vi "HXG2_Fluid-Averages.vi"(8 "error in (no error)":errorcluster, 9 "Analog DATA In":T3, 10 "BoolSelection In":T2, 11 "CalcValues":T1) -> (0 "error out":errorcluster, 3 "Calculated Values":T1)   [LabVIEW 2012]
doc: "This VI will average all air side and glycol side input temperatures based on boolean selections of what sensors to use."
uses:
  Controls/HXG2_Calculated.ctl
  Controls/HXG2_AnalogIn.ctl
  Controls/HXG2_BooleanSelections.ctl
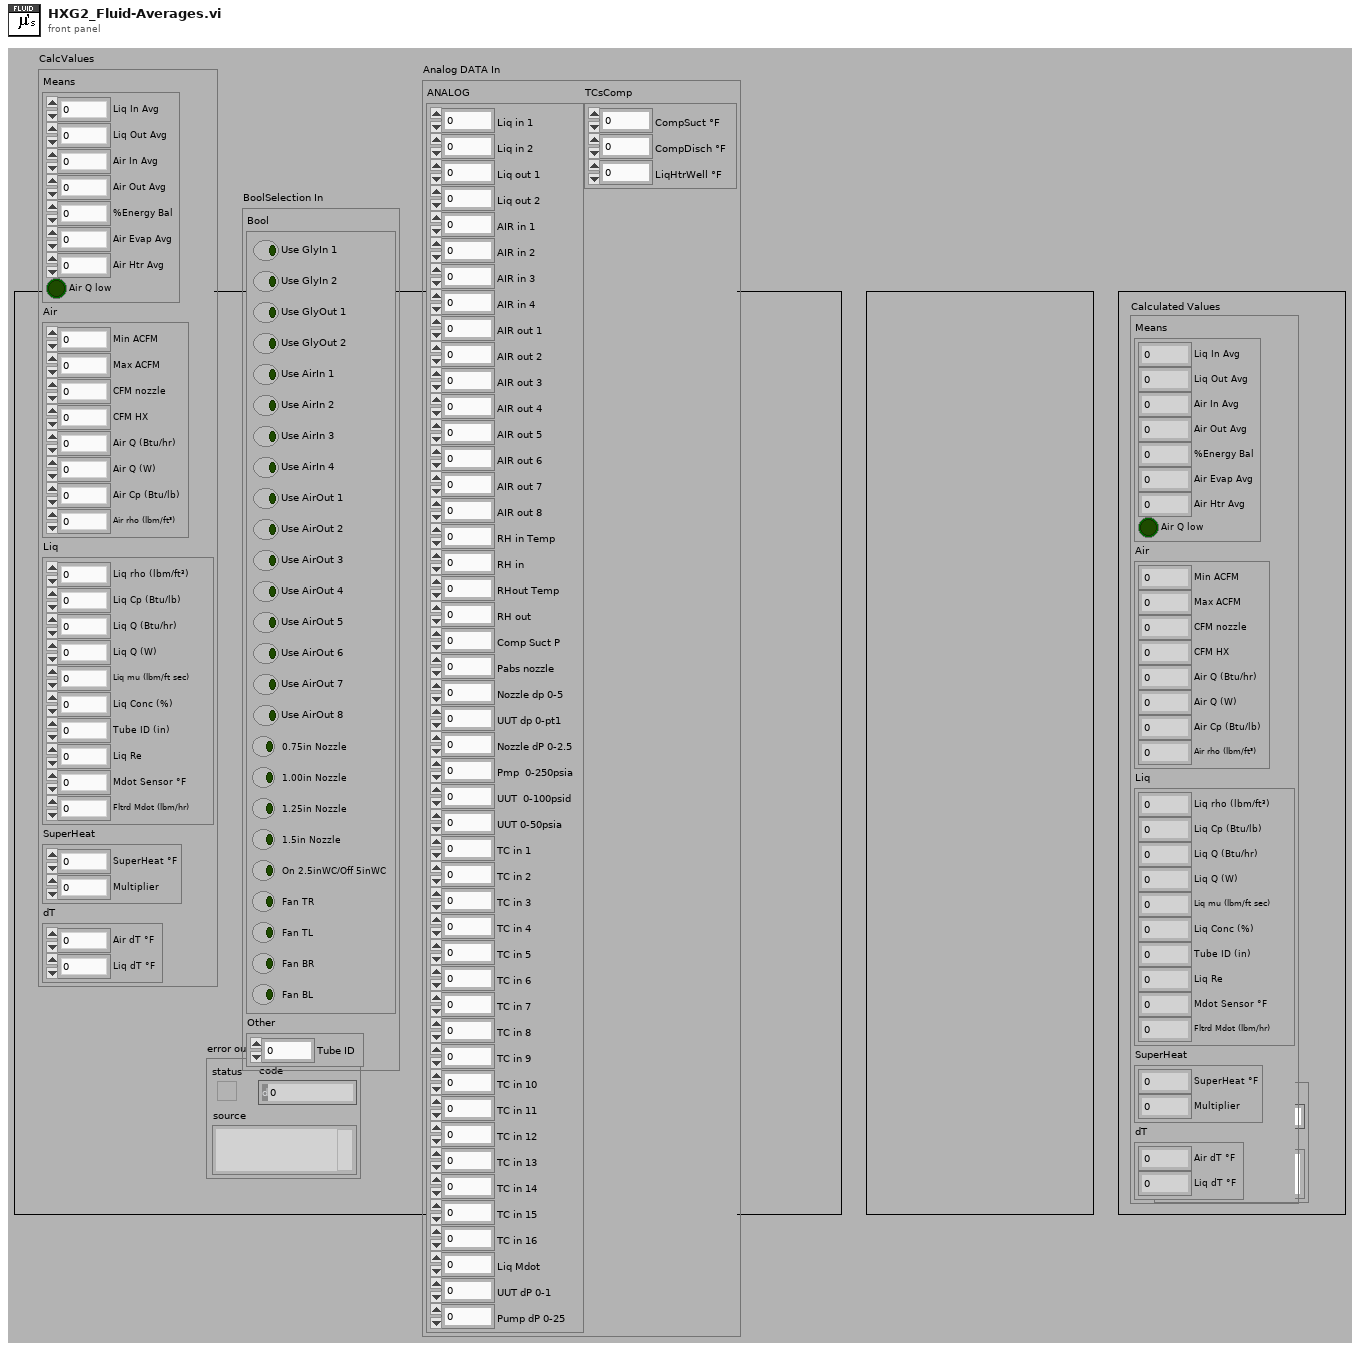
[diagram p1: front panel]
types:
  T1 = typedef "HXG2_Calculated.ctl" = cluster{"Means":cluster{"Liq In Avg":dbl, "Liq Out Avg":dbl, "Air In Avg":dbl, "Air Out Avg":dbl, "%Energy Bal":dbl, "Air Evap Avg":dbl, "Air Htr Avg":dbl, "Air Q low":bool}, "Air":cluster{"Min ACFM":dbl, "Max ACFM":dbl, "CFM nozzle":dbl, "CFM HX":dbl, "Air Q (Btu/hr)":dbl, "Air Q (W)":dbl, "Air Cp (Btu/lb)":dbl, "Air rho (lbm/ft³)":dbl}, "Liq":cluster{"Liq rho (lbm/ft³)":dbl, "Liq Cp (Btu/lb)":dbl, "Liq Q (Btu/hr)":dbl, "Liq Q (W)":dbl, "Liq mu (lbm/ft sec)":dbl, "Liq Conc (%)":dbl, "Tube ID (in)":dbl, "Liq Re":dbl, "Mdot Sensor °F":dbl, "Fltrd Mdot (lbm/hr)":dbl}, "SuperHeat":cluster{"SuperHeat °F":dbl, "Multiplier":dbl}, "dT":cluster{"Air dT °F":dbl, "Liq dT °F":dbl}}
  T2 = typedef "HXG2_BooleanSelections.ctl" = cluster{"Bool":cluster{"Use GlyIn 1":bool, "Use GlyIn 2":bool, "Use GlyOut 1":bool, "Use GlyOut 2":bool, "Use AirIn 1":bool, "Use AirIn 2":bool, "Use AirIn 3":bool, "Use AirIn 4":bool, "Use AirOut 1":bool, "Use AirOut 2":bool, "Use AirOut 3":bool, "Use AirOut 4":bool, "Use AirOut 5":bool, "Use AirOut 6":bool, "Use AirOut 7":bool, "Use AirOut 8":bool, "0.75in Nozzle":bool, "1.00in Nozzle":bool, "1.25in Nozzle":bool, "1.5in Nozzle":bool, "On 2.5inWC/Off 5inWC":bool, "Fan TR":bool, "Fan TL":bool, "Fan BR":bool, "Fan BL":bool}, "Other":cluster{"Tube ID":dbl}}
  T3 = typedef "HXG2_AnalogIn.ctl" = cluster{"ANALOG":cluster{"Liq in 1":dbl, "Liq in 2":dbl, "Liq out 1":dbl, "Liq out 2":dbl, "AIR in 1":dbl, "AIR in 2":dbl, "AIR in 3":dbl, "AIR in 4":dbl, "AIR out 1":dbl, "AIR out 2":dbl, "AIR out 3":dbl, "AIR out 4":dbl, "AIR out 5":dbl, "AIR out 6":dbl, "AIR out 7":dbl, "AIR out 8":dbl, "RH in Temp":dbl, "RH in":dbl, "RHout Temp":dbl, "RH out":dbl, "Comp Suct P":dbl, "Pabs nozzle":dbl, "Nozzle dp 0-5":dbl, "UUT dp 0-pt1":dbl, "Nozzle dP 0-2.5":dbl, "Pmp  0-250psia":dbl, "UUT  0-100psid":dbl, "UUT 0-50psia":dbl, "TC in 1":dbl, "TC in 2":dbl, "TC in 3":dbl, "TC in 4":dbl, "TC in 5":dbl, "TC in 6":dbl, "TC in 7":dbl, "TC in 8":dbl, "TC in 9":dbl, "TC in 10":dbl, "TC in 11":dbl, "TC in 12":dbl, "TC in 13":dbl, "TC in 14":dbl, "TC in 15":dbl, "TC in 16":dbl, "Liq Mdot":dbl, "UUT dP 0-1":dbl, "Pump dP 0-25":dbl}, "TCsComp":cluster{"CompSuct °F  ":dbl, "CompDisch °F":dbl, "LiqHtrWell °F":dbl}}
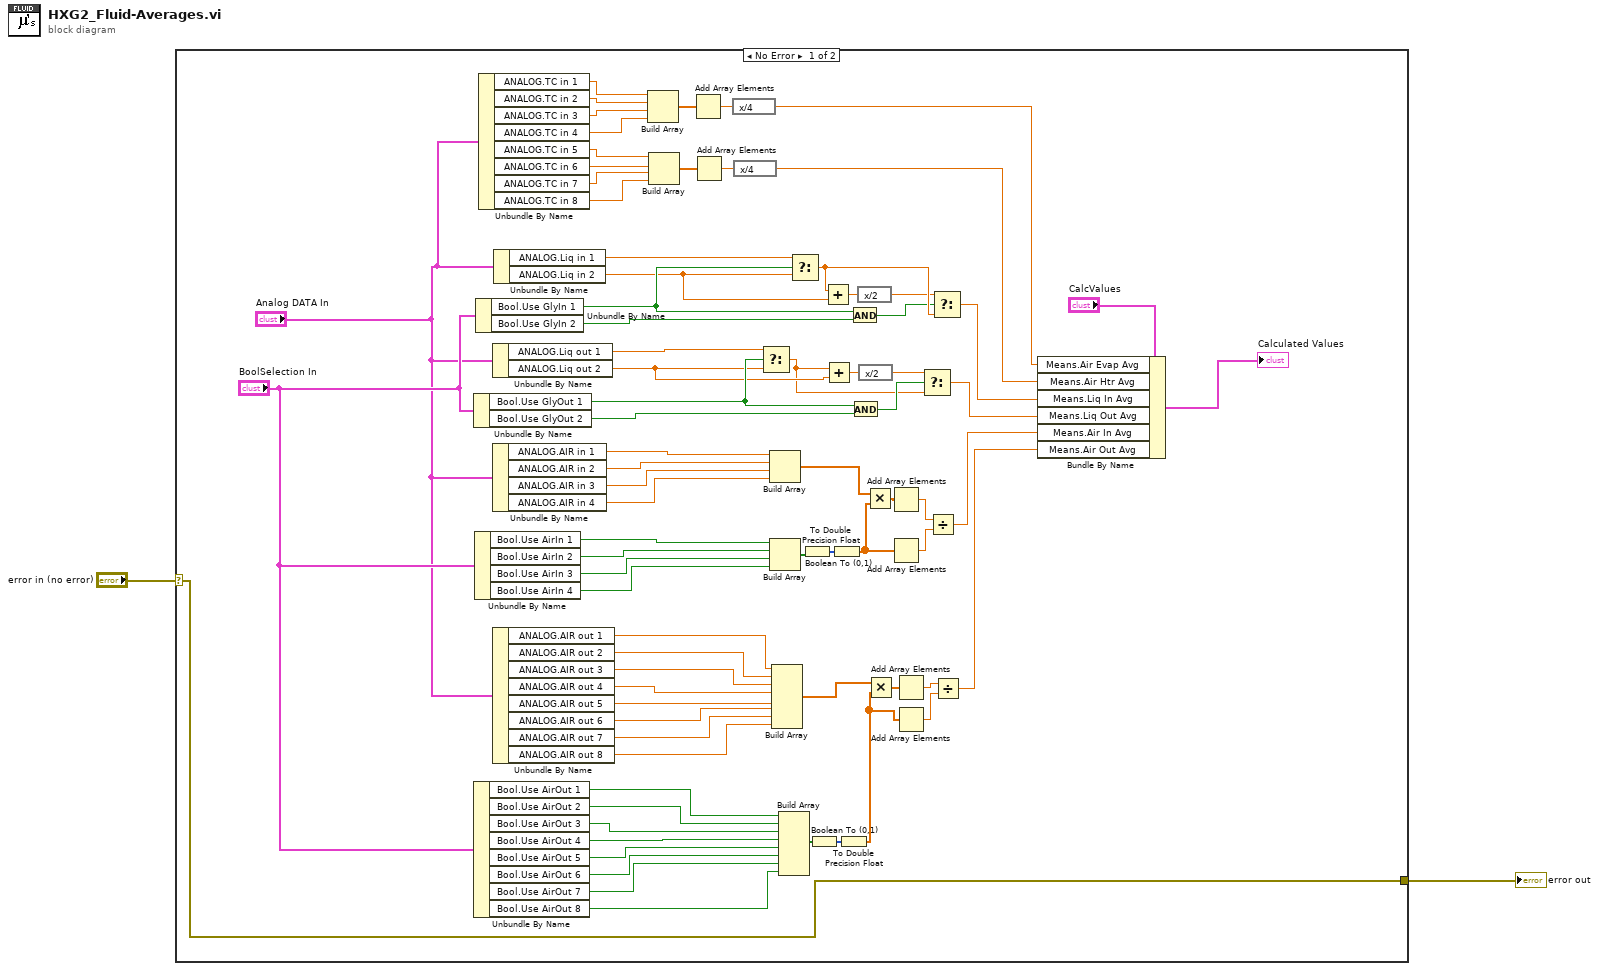
[diagram p0: block diagram]
diagram:
  n1 = case shown="No Error" "error in (no error)" {
    selector: "error in (no error)" -> [w18 w80]
    tunnel: [w18 w80] -> w1
    frame No Error {
      n2 = Unbundle By Name("BoolSelection In") -> ("Bool.Use GlyOut 1"=w36:bool, "Bool.Use GlyOut 2"=w37:bool)
      n3 = Unbundle By Name("BoolSelection In") -> ("Bool.Use AirOut 1"=w66:bool, "Bool.Use AirOut 2"=w65:bool, "Bool.Use AirOut 3"=w64:bool, "Bool.Use AirOut 4"=w63:bool, "Bool.Use AirOut 5"=w76:bool, "Bool.Use AirOut 6"=w77:bool, "Bool.Use AirOut 7"=w78:bool, "Bool.Use AirOut 8"=w79:bool)
      n4 = Unbundle By Name("BoolSelection In") -> ("Bool.Use AirIn 1"=w44:bool, "Bool.Use AirIn 2"=w45:bool, "Bool.Use AirIn 3"=w46:bool, "Bool.Use AirIn 4"=w47:bool)
      n5 = Unbundle By Name("BoolSelection In") -> ("Bool.Use GlyIn 1"=w28:bool, "Bool.Use GlyIn 2"=w29:bool)
      n6 = Unbundle By Name("Analog DATA In") -> ("ANALOG.TC in 1"=w16:dbl, "ANALOG.TC in 2"=w15:dbl, "ANALOG.TC in 3"=w14:dbl, "ANALOG.TC in 4"=w13:dbl, "ANALOG.TC in 5"=w7:dbl, "ANALOG.TC in 6"=w6:dbl, "ANALOG.TC in 7"=w5:dbl, "ANALOG.TC in 8"=w4:dbl)
      n7 = Unbundle By Name("Analog DATA In") -> ("ANALOG.Liq out 1"=w34:dbl, "ANALOG.Liq out 2"=w35:dbl)
      n8 = Unbundle By Name("Analog DATA In") -> ("ANALOG.AIR in 1"=w40:dbl, "ANALOG.AIR in 2"=w41:dbl, "ANALOG.AIR in 3"=w42:dbl, "ANALOG.AIR in 4"=w43:dbl)
      n9 = Unbundle By Name("Analog DATA In") -> ("ANALOG.AIR out 1"=w70:dbl, "ANALOG.AIR out 2"=w69:dbl, "ANALOG.AIR out 3"=w68:dbl, "ANALOG.AIR out 4"=w67:dbl, "ANALOG.AIR out 5"=w71:dbl, "ANALOG.AIR out 6"=w72:dbl, "ANALOG.AIR out 7"=w73:dbl, "ANALOG.AIR out 8"=w74:dbl)
      n10 = Unbundle By Name("Analog DATA In") -> ("ANALOG.Liq in 1"=w24:dbl, "ANALOG.Liq in 2"=w26:dbl)
      n11 = Build Array(w16, w15, w14, w13) -> (w12:dbl[])
      n12 = Build Array(w7, w6, w5, w4) -> (w8:dbl[])
      n13 = Add Array Elements(numeric array=w12) -> (sum=w11:dbl)
      n14 = Add Array Elements(numeric array=w8) -> (sum=w9:dbl)
      n15 = expression code="x/4"(w11) -> (w10:dbl)
      n16 = expression code="x/4"(w9) -> (w3:dbl)
      n17 = Select(t=w34, s=w36, f=w35) -> (s? t:f=w30:dbl)
      n18 = Build Array(w40, w41, w42, w43) -> (w50:dbl[])
      n19 = Build Array(w44, w45, w46, w47) -> (w49:bool[])
      n20 = Build Array(w70, w69, w68, w67, w71, w72, w73, w74) -> (w60:dbl[])
      n21 = Build Array(w66, w65, w64, w63, w76, w77, w78, w79) -> (w61:bool[])
      n22 = Select(t=w24, s=w28, f=w26) -> (s? t:f=w27:dbl)
      n23 = Boolean To (0,1)(Boolean=w49) -> (0, 1=w48:i16[])
      n24 = Boolean To (0,1)(Boolean=w61) -> (0, 1=w62:i16[])
      n25 = Add(x=w27, y=w26) -> (x+y=w23:dbl)
      n26 = Add(x=w30, y=w35) -> (x+y=w32:dbl)
      n27 = To Double Precision Float(number=w48) -> (double precision float=w52:dbl[])
      n28 = To Double Precision Float(number=w62) -> (double precision float=w58:dbl[])
      n29 = And(x=w28, y=w29) -> (x .and. y?=w22:bool)
      n30 = And(x=w36, y=w37) -> (x .and. y?=w33:bool)
      n31 = expression code="x/2"(w23) -> (w25:dbl)
      n32 = expression code="x/2"(w32) -> (w31:dbl)
      n33 = Multiply(x=w50, y=w52) -> (x*y=w51:dbl[])
      n34 = Multiply(x=w60, y=w58) -> (x*y=w59:dbl[])
      n35 = Add Array Elements(numeric array=w51) -> (sum=w54:dbl)
      n36 = Add Array Elements(numeric array=w52) -> (sum=w53:dbl)
      n37 = Add Array Elements(numeric array=w59) -> (sum=w56:dbl)
      n38 = Add Array Elements(numeric array=w58) -> (sum=w57:dbl)
      n39 = Select(t=w31, s=w33, f=w30) -> (s? t:f=w39:dbl)
      n40 = Divide(x=w54, y=w53) -> (x/y=w55:dbl)
      n41 = Select(t=w25, s=w22, f=w27) -> (s? t:f=w38:dbl)
      n42 = Divide(x=w56, y=w57) -> (x/y=w75:dbl)
      n43 = Bundle By Name(cluster="CalcValues", "Means.Air Evap Avg"=w10, "Means.Air Htr Avg"=w3, "Means.Liq In Avg"=w38, "Means.Liq Out Avg"=w39, "Means.Air In Avg"=w55, "Means.Air Out Avg"=w75) -> (→"Calculated Values":T1)
    }
    frame Error {
    }
  }
  "error out" <- w1
